vi "Monitor.vi"(0 "object in":refnum<class "MTec.lvclass">, 5 "error in (no error)":errorcluster) -> (14 "object out":refnum<class "MTec.lvclass">, 16 "MtecData":T3={"meTEC_CH2_Temperature Stability"=1, "meTEC_CH2_Act. Output Current [A]"=0.0, "meTEC_CH2_Act. Output Voltage [V]"=0.0, "meTEC_CH2_Object Temperature [°C]"=0.0, "meTEC_CH2_Sink Temperature [°C]"=0.0, "meTEC_CH1_Error Parameter"=0, "meTEC_CH1_Error Instance"=0, "meTEC_CH1_Error No."=0, "meTEC_CH1_Device Status"=1, "meTEC_CH1_Temperature Stability"=1, "meTEC_CH1_Act. Output Current [A]"=0.0, "meTEC_CH1_Act. Output Voltage [V]"=0.0, "meTEC_CH1_Object Temperature [°C]"=0.0, "meTEC_CH1_Sink Temperature [°C]"=0.0} {"meTEC_CH1_Sink Temperature [°C]" format="%.3f"; "meTEC_CH1_Object Temperature [°C]" format="%.3f"; "meTEC_CH1_Act. Output Voltage [V]" format="%.3f"; "meTEC_CH1_Act. Output Current [A]" format="%.3f"; "meTEC_CH1_Temperature Stability" items=["Temperature regulation is not active", "Is not stable", "Is stable"]; "meTEC_CH1_Device Status" items=["Initializing", "Ready", "Run", "Error", "Bootloader", "Reset in Progress"]; "meTEC_CH2_Sink Temperature [°C]" format="%.3f"; "meTEC_CH2_Object Temperature [°C]" format="%.3f"; "meTEC_CH2_Act. Output Voltage [V]" format="%.3f"; "meTEC_CH2_Act. Output Current [A]" format="%.3f"; "meTEC_CH2_Temperature Stability" items=["Temperature regulation is not active", "Is not stable", "Is stable"]}, 19 "error out":errorcluster)   [LabVIEW 2019, in "MTec.lvclass"]
uses:
  MTec.lvclass
  TEC LabVIEW Control Software v0.14/Source/LV Source/[meerstetter engineering TE Cooling]/TypeDefs/meTEC_ID 1200_Temperature is Stable.ctl
  TEC LabVIEW Control Software v0.14/Source/LV Source/[meerstetter engineering TE Cooling]/TypeDefs/meTEC_ID 104_Device Status.ctl
  MTec.lvclass/MTec.ctl
panel:
  out "meTEC_CH1_Sink Temperature [°C]":dbl caption="Sink Temperature [°C]" format="%.3f"
  out "meTEC_CH1_Object Temperature [°C]":dbl caption="Object Temperature [°C]" format="%.3f"
  out "meTEC_CH1_Act. Output Voltage [V]":dbl caption="Act. Output Voltage [V]" format="%.3f"
  out "meTEC_CH1_Act. Output Current [A]":dbl caption="Act. Output Current [A]" format="%.3f"
  out "meTEC_CH1_Temperature Stability":T1=1 caption="Temperature Stabilty" items=["Temperature regulation is not active", "Is not stable", "Is stable"]
  out "meTEC_CH1_Device Status":T2=1 caption="Device Status" items=["Initializing", "Ready", "Run", "Error", "Bootloader", "Reset in Progress"]
  out "meTEC_CH1_Error No.":i32 caption="Error No."
  out "meTEC_CH1_Error Instance":i32 caption="Error Instance"
  out "meTEC_CH1_Error Parameter":i32 caption="Error Parameter"
  out "meTEC_CH2_Sink Temperature [°C]":dbl caption="Sink Temperature [°C]" format="%.3f"
  out "meTEC_CH2_Object Temperature [°C]":dbl caption="Object Temperature [°C]" format="%.3f"
  out "meTEC_CH2_Act. Output Voltage [V]":dbl caption="Act. Output Voltage [V]" format="%.3f"
  out "meTEC_CH2_Act. Output Current [A]":dbl caption="Act. Output Current [A]" format="%.3f"
  out "meTEC_CH2_Temperature Stability":T1=1 caption="Temperature Stabilty" items=["Temperature regulation is not active", "Is not stable", "Is stable"]
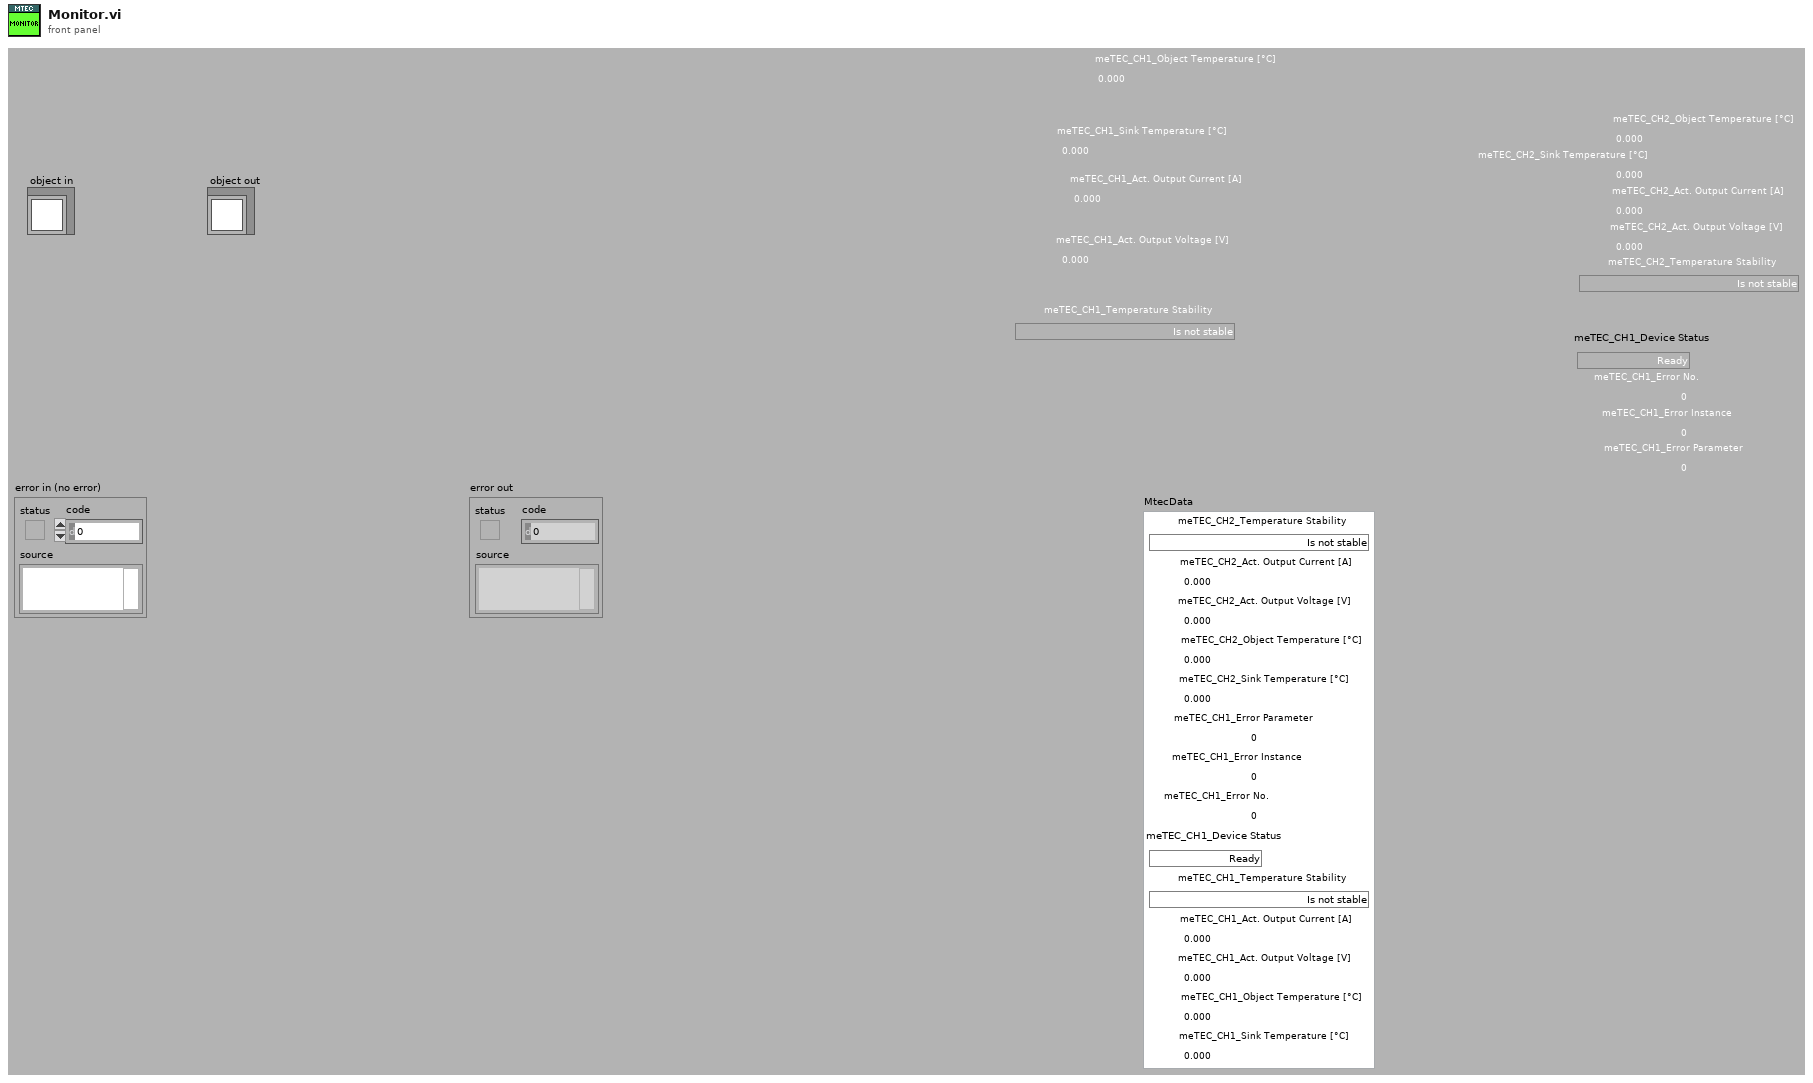
[diagram p1: front panel]
types:
  T1 = typedef "meTEC_ID 1200_Temperature is Stable.ctl" = i32
  T2 = typedef "meTEC_ID 104_Device Status.ctl" = i32
  T3 = cluster{"meTEC_CH2_Temperature Stability":T1, "meTEC_CH2_Act. Output Current [A]":dbl, "meTEC_CH2_Act. Output Voltage [V]":dbl, "meTEC_CH2_Object Temperature [°C]":dbl, "meTEC_CH2_Sink Temperature [°C]":dbl, "meTEC_CH1_Error Parameter":i32, "meTEC_CH1_Error Instance":i32, "meTEC_CH1_Error No.":i32, "meTEC_CH1_Device Status":T2, "meTEC_CH1_Temperature Stability":T1, "meTEC_CH1_Act. Output Current [A]":dbl, "meTEC_CH1_Act. Output Voltage [V]":dbl, "meTEC_CH1_Object Temperature [°C]":dbl, "meTEC_CH1_Sink Temperature [°C]":dbl}
  T4 = typedef "FGV_TE Controller.ctl" = cluster{"SVs":cluster{"Unused":dbl}, "PVs":cluster{"FW & HW Versions":cluster{"Device Type [I32]":i32, "Device Type [String]":string, "Firmware Version [I32]":i32, "Firmware Version [String]":string, "Hardware Version [I32]":i32, "Hardware Version [String]":string, "Serial No.":i32}, "TEC Configuration":T5, "Object Target Temperature Source_CH1":u8, "Object Target Temperature Source_CH2":u8}, "Front Panel References":T6}
  T5 = typedef "meTEC_Configuration.ctl" = cluster{"VISA resource name":refnum<visa-resource-name>, "Device Address":u16}
  T6 = typedef "FGV_Front Panel References.ctl" = cluster{"Main Loop Queue":refnum<queue>, "meTEC_Device Type":refnum<vi>, "meTEC_Serial No.":refnum<vi>, "meTEC_Hardware Version":refnum<vi>, "meTEC_Firmware Version":refnum<vi>, "meTEC_CH1_Object Target Temperature (ID 3000 / 50012) [°C]":refnum<vi>, "meTEC_CH1_Live Set Current (ID 50001) [A]":refnum<vi>, "meTEC_CH1_Live Set Voltage (ID 50002) [V]":refnum<vi>, "meTEC_CH1_Live Enable (ID 50000)":refnum<vi>, "meTEC_CH1_Input Selection (ID 2000)":refnum<vi>, "meTEC_CH1_Object Target Temp. Source Sel. (ID 50011)":refnum<vi>, "meTEC_CH2_Object Target Temperature (ID 3000 / 50012) [°C]":refnum<vi>, "meTEC_CH2_Live Set Current (ID 50001) [A]":refnum<vi>, "meTEC_CH2_Live Set Voltage (ID 50002) [V]":refnum<vi>, "meTEC_CH2_Live Enable (ID 50000)":refnum<vi>, "meTEC_CH2_Input Selection (ID 2000)":refnum<vi>, "meTEC_CH2_Object Target Temp. Source Sel. (ID 50011)":refnum<vi>, "meTEC_CH2_Object Temperature [°C]":refnum<vi>, "meTEC_CH2_Sink Temperature [°C]":refnum<vi>, "meTEC_CH2_Act. Output Current [A]":refnum<vi>, "meTEC_CH2_Act. Output Voltage [V]":refnum<vi>, "meTEC_CH2_Temperature Stability":refnum<vi>, "Monitor Chart_CH2":refnum<vi>, "meTEC_Initialize Device":refnum<vi>}
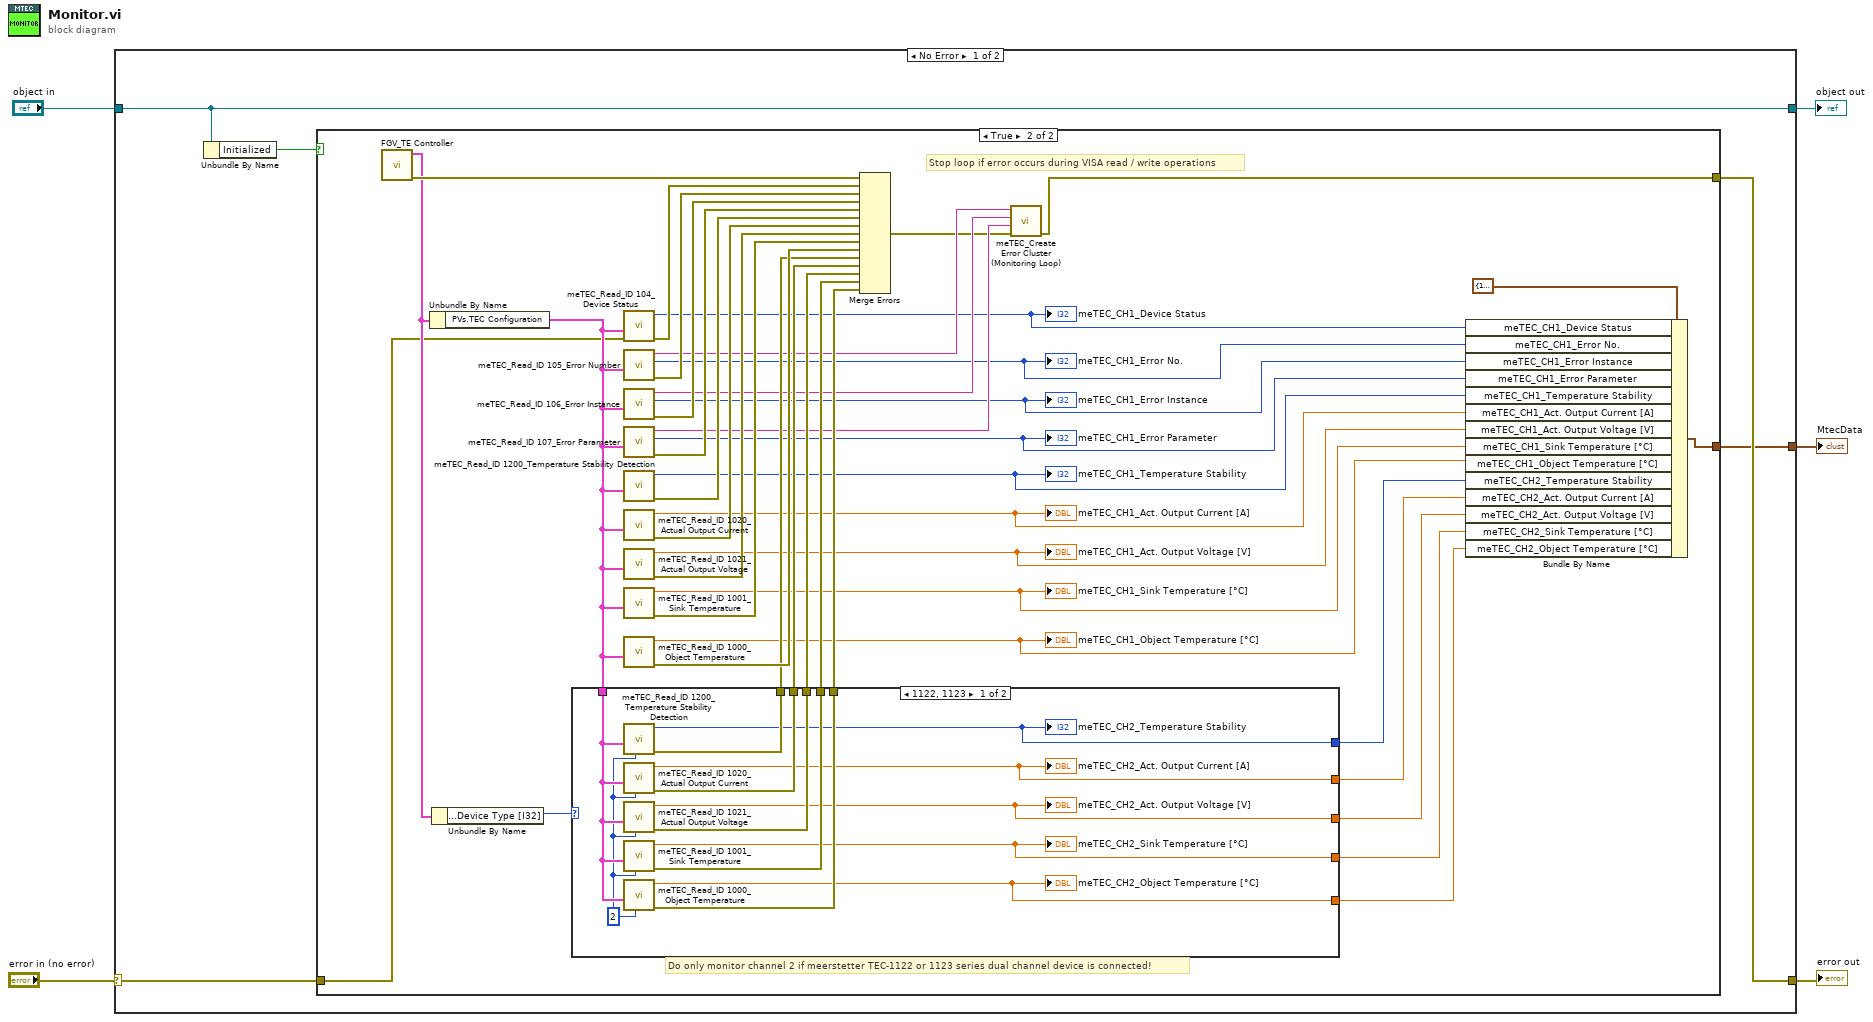
[diagram p0: block diagram]
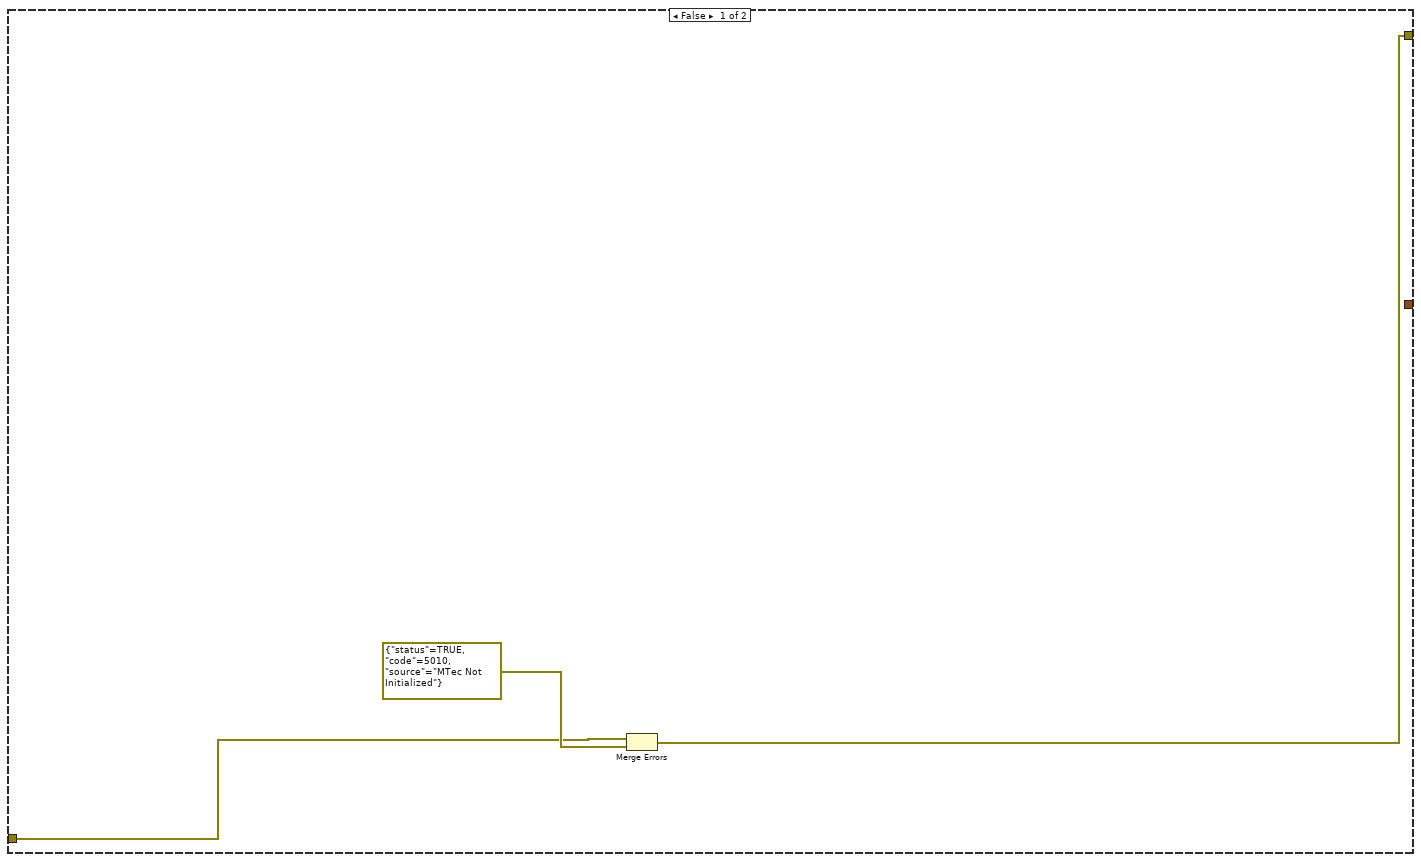
[diagram p2: hidden frame]
diagram:
  n1 = case shown="No Error" "error in (no error)" {
    selector: "error in (no error)" -> [w9 w67]
    tunnel: [w8 w67] -> w4
    tunnel: [w10 w66] -> w2
    tunnel: "object in" -> [w10 w66]
    tunnel: [w7 _] -> w1
    frame No Error {
      n2 = Unbundle By Name(w10) -> ("Initialized"=w6:bool)
      n3 = case shown="True" w6 {
        tunnel: w9 -> [w12 w16]
        tunnel: [w11 w15] -> w8
        tunnel: [_ w14] -> w7
        frame False {
          n4 = Merge Errors(w12, errorcluster {"status"=TRUE, "code"=5010, "source"="MTec Not Initialized"} ("error in (no error)")) -> (w11:errorcluster)
        }
        frame True {
          # "Do only monitor channel 2 if meerstetter TEC-1122 or 1123 series dual channel device is connected!"
          # "Stop loop if error occurs during VISA read / write operations"
          n5 = call "FGV_TE Controller.vi"() -> ("error out"=w53:errorcluster, "FGV_TEC_OUT"=w38:T4)  [unwired: 10 in]
          n6 = Unbundle By Name(w38) -> ("PVs.TEC Configuration"=w36:T5)
          n7 = Unbundle By Name(w38) -> ("PVs.FW & HW Versions.Device Type [I32]"=w37:i32)
          n8 = case shown="1122, 1123" w37 {
            tunnel: w36 -> [w65 _]
            tunnel: [w64 _] -> w43
            tunnel: [w63 _] -> w42
            tunnel: [w62 _] -> w41
            tunnel: [w61 _] -> w40
            tunnel: [w60 _] -> w39
            tunnel: [w58 _] -> w21
            tunnel: [w57 _] -> w20
            tunnel: [w56 _] -> w19
            tunnel: [w55 _] -> w18
            tunnel: [w54 _] -> w17
            frame 1122, 1123 {
              w59 = u8 2 ("Instance (1)")
              n9 = call "meTEC_Read_ID 1200_Temperature Stability Detection.vi"("Instance (1)"=w59, "TEC Configuration_IN"=w65) -> ("error out"=w64:errorcluster, "Temperature is Stable? [I32)] (ID 1200)"=w58:i32)  [unwired: 6 in, 2 out]
              "meTEC_CH2_Temperature Stability" <- w58
              n10 = call "meTEC_Read_ID 1020_Actual Output Current.vi"("Instance (1)"=w59, "TEC Configuration_IN"=w65) -> ("error out"=w63:errorcluster, "Act. Output Current [A] (ID 1020)"=w57:dbl)  [unwired: 7 in, 1 out]
              "meTEC_CH2_Act. Output Current [A]" <- w57
              n11 = call "meTEC_Read_ID 1021_Actual Output Voltage.vi"("Instance (1)"=w59, "TEC Configuration_IN"=w65) -> ("error out"=w62:errorcluster, "Act. Output Voltage [A] (ID 1021)"=w56:dbl)  [unwired: 7 in, 1 out]
              "meTEC_CH2_Act. Output Voltage [V]" <- w56
              n12 = call "meTEC_Read_ID 1001_Sink Temperature.vi"("Instance (1)"=w59, "TEC Configuration_IN"=w65) -> ("error out"=w61:errorcluster, "Sink Temperature [°C] (ID 1001)"=w55:dbl)  [unwired: 7 in, 1 out]
              "meTEC_CH2_Sink Temperature [°C]" <- w55
              n13 = call "meTEC_Read_ID 1000_Object Temperature.vi"("Instance (1)"=w59, "TEC Configuration_IN"=w65) -> ("error out"=w60:errorcluster, "Object Temperature [°C] (ID 1000)"=w54:dbl)  [unwired: 7 in, 1 out]
              "meTEC_CH2_Object Temperature [°C]" <- w54
            }
            frame 1089..1091, Default {
            }
          }
          n14 = call "meTEC_Read_ID 104_Device Status.vi"("error in (no error)"=w16, "TEC Configuration_IN"=w36) -> ("error out"=w47:errorcluster, "Device Status (ID 104) [I32]"=w30:i32)  [unwired: 7 in, 1 out]
          "meTEC_CH1_Device Status" <- w30
          n15 = call "meTEC_Read_ID 105_Error Number.vi"("TEC Configuration_IN"=w36) -> ("error out"=w46:errorcluster, "Error Number (ID 105) [I32]"=w29:i32, "Error Number (ID 105) [String]"=w33:string)  [unwired: 7 in, 1 out]
          "meTEC_CH1_Error No." <- w29
          n16 = call "meTEC_Read_ID 106_Error Instance.vi"("TEC Configuration_IN"=w36) -> ("error out"=w45:errorcluster, "Error Instance (ID 106) [I32]"=w28:i32, "Error Instance (ID 106) [String]"=w34:string)  [unwired: 7 in, 1 out]
          "meTEC_CH1_Error Instance" <- w28
          n17 = call "meTEC_Read_ID 107_Error Parameter.vi"("TEC Configuration_IN"=w36) -> ("error out"=w44:errorcluster, "Error Parameter (ID 107) [I32]"=w27:i32, "Error Parameter (ID 107) [String]"=w35:string)  [unwired: 7 in, 1 out]
          "meTEC_CH1_Error Parameter" <- w27
          n18 = call "meTEC_Read_ID 1200_Temperature Stability Detection.vi"("TEC Configuration_IN"=w36) -> ("error out"=w52:errorcluster, "Temperature is Stable? [I32)] (ID 1200)"=w26:i32)  [unwired: 7 in, 2 out]
          "meTEC_CH1_Temperature Stability" <- w26
          n19 = call "meTEC_Read_ID 1020_Actual Output Current.vi"("TEC Configuration_IN"=w36) -> ("error out"=w51:errorcluster, "Act. Output Current [A] (ID 1020)"=w25:dbl)  [unwired: 8 in, 1 out]
          "meTEC_CH1_Act. Output Current [A]" <- w25
          n20 = call "meTEC_Read_ID 1021_Actual Output Voltage.vi"("TEC Configuration_IN"=w36) -> ("error out"=w50:errorcluster, "Act. Output Voltage [A] (ID 1021)"=w24:dbl)  [unwired: 8 in, 1 out]
          "meTEC_CH1_Act. Output Voltage [V]" <- w24
          n21 = call "meTEC_Read_ID 1001_Sink Temperature.vi"("TEC Configuration_IN"=w36) -> ("error out"=w49:errorcluster, "Sink Temperature [°C] (ID 1001)"=w23:dbl)  [unwired: 8 in, 1 out]
          "meTEC_CH1_Sink Temperature [°C]" <- w23
          n22 = call "meTEC_Read_ID 1000_Object Temperature.vi"("TEC Configuration_IN"=w36) -> ("error out"=w48:errorcluster, "Object Temperature [°C] (ID 1000)"=w22:dbl)  [unwired: 8 in, 1 out]
          "meTEC_CH1_Object Temperature [°C]" <- w22
          n23 = Merge Errors(w53, w47, w46, w45, w44, w52, w51, w50, w49, w48, w43, w42, w41, w40, w39) -> (w32:errorcluster)
          n24 = call "meTEC_Create Error Cluster (Monitoring Loop).vi"("error in (no error)"=w32, "Error Parameter"=w35, "Error Instance"=w34, "Error Number"=w33) -> ("error out"=w15:errorcluster)  [unwired: 7 in]
          n25 = Bundle By Name(cluster=T3 {"meTEC_CH2_Temperature Stability"=1, "meTEC_CH2_Act. Output Current [A]"=0.0, "meTEC_CH2_Act. Output Voltage [V]"=0.0, "meTEC_CH2_Object Temperature [°C]"=0.0, "meTEC_CH2_Sink Temperature [°C]"=0.0, "meTEC_CH1_Error Parameter"=0, "meTEC_CH1_Error Instance"=0, "meTEC_CH1_Error No."=0, "meTEC_CH1_Device Status"=1, "meTEC_CH1_Temperature Stability"=1, "meTEC_CH1_Act. Output Current [A]"=0.0, "meTEC_CH1_Act. Output Voltage [V]"=0.0, "meTEC_CH1_Object Temperature [°C]"=0.0, "meTEC_CH1_Sink Temperature [°C]"=0.0} ("Cluster"), "meTEC_CH1_Device Status"=w30, "meTEC_CH1_Error No."=w29, "meTEC_CH1_Error Instance"=w28, "meTEC_CH1_Error Parameter"=w27, "meTEC_CH1_Temperature Stability"=w26, "meTEC_CH1_Act. Output Current [A]"=w25, "meTEC_CH1_Act. Output Voltage [V]"=w24, "meTEC_CH1_Sink Temperature [°C]"=w23, "meTEC_CH1_Object Temperature [°C]"=w22, "meTEC_CH2_Temperature Stability"=w21, "meTEC_CH2_Act. Output Current [A]"=w20, "meTEC_CH2_Act. Output Voltage [V]"=w19, "meTEC_CH2_Sink Temperature [°C]"=w18, "meTEC_CH2_Object Temperature [°C]"=w17) -> (w14:T3)
        }
      }
    }
    frame Error {
    }
  }
  "error out" <- w4
  "object out" <- w2
  "MtecData" <- w1
